vi "AlliGator Define & Save Intensity Corrections File.vi"() -> ()   [LabVIEW 2021, in "AlliGator Intensity Corrections.lvlib"]
doc: "UI to enter intensity correction sepcifications."
uses:
  AlliGator Intensity Corrections.lvlib
  AlliGator Q Element.ctl
  AlliGator Q Event.ctl
  <vilib>/Utility/file.llb/Write Delimited Spreadsheet (DBL).vi
  AlliGator Action Engine.lvlib
panel:
  in  "Save Correction File":bool
  in  "Check Corrections":bool
  out "Intensity Correction":dbl[](graph)
  in  "Acquisition Parameters":string[][](table)=[["1", "1", "550", "200", "250"], ["5", "0.9", "", "", ""], ["15", "0.8", "", "", ""], ["22", "0.7", "", "", ""], ["40", "", "", "", ""], ["53", "", "", "", ""], ["57", "0.6", "", "", ""], ["67", "", "", "", ""], ["73", "", "", "", ""], ["77", "", "", "", ""]]
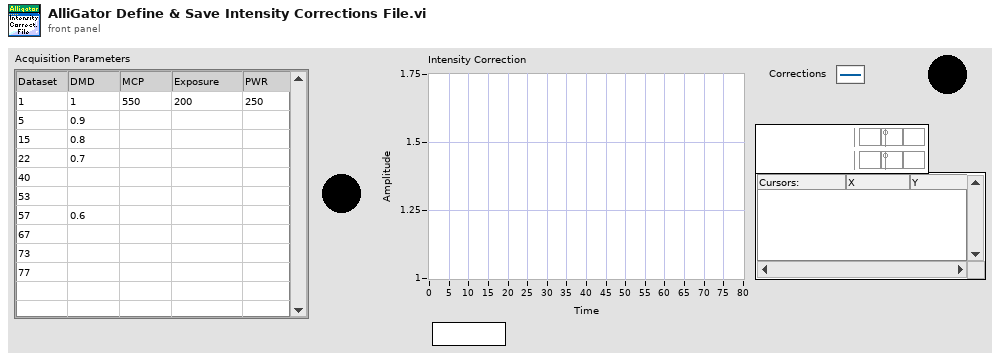
[diagram p1: front panel]
types:
  T1 = typedef "AlliGator Action Engine.lvlib/AlliGator Q Element.ctl" = cluster{"AlliGator Q Event":T2, "Data":variant}
  T2 = typedef "AlliGator Action Engine.lvlib/AlliGator Q Event.ctl" = enum16{"---- Files ----", "Files:Set Batch Export Files To Save", "Files:Set Dataset Loading & Pre-processing Options", "Files:Check #Frames in Dataset", "Files:Increment Frame Index", "Files:Open Mask Image", "Files:Open White Light Image", "Files:Open Single Dataset", "Files:New Folder of Folders Selected", "Files:Load File (all Types)_Scriptable", "Files:Move Flattened Series to Folders Series", "Files:Select Folder", "Files:Load FLI Dataset", "Files:Load Swiss SPAD 1 Dataset", "Files:Load Swiss SPAD 2 Dataset", "Files:Load .sdt FLI Dataset", "Files:Load .ptu FLI Dataset", "Files:Load .bin FLI Dataset", "Files:Load Single Gate Image Folder", "Files:Load I/m/phi Dataset (deprecated)", "Files:Load Single Image", "Files:Subtract Background File", "Files:Export FLI Dataset", "Files:Load HDF5 FLI Dataset", "Files:Set Destination File Path", "Files:Save Mask Image", "Files:Batch Conversion", "Files:New Folder Selected", "Files:Close FLI Dataset", "Files:Close FLI Dataset Series", "Files:Close White Light Image", "Files:Close Mask Image", "---- FLI Dataset ----", "FLI Dataset:Channel Arithmetic", "FLI Dataset:Export Average Lifetime Map as ASCII", "FLI Dataset:Export User-Defined Quantity Map as ASCII", "FLI Dataset:Python Function FLI Dataset Event", "FLI Dataset:ROI Analysis", "FLI Dataset:Tilted Logistic Square Gated IRF Characteristics Map", "FLI Dataset:Logistic Square Gated IRF Characteristics Map", "FLI Dataset:Square Gated IRF Characteristics Map", "FLI Dataset:Multi-ROI Single-Pixel Phasor Analysis", "FLI Dataset:Multi-ROI Single-Pixel NLSF Analysis", "FLI Dataset:All ROIs IRF Extraction", "FLI Dataset:All ROIs Decay Fit Non-Interactive (Fast + Individual IRF)", "FLI Dataset:All ROIs Phasor Analysis", "FLI Dataset:All ROIs Decay Fit", "FLI Dataset:Fluorescence Decay Statistics", "FLI Dataset:Update Decay Statistics Graph", "FLI Dataset:Get Decay from ROI", "FLI Dataset:All ROIs Average Lifetimes", "---- FLI Dataset Series ----", "FLI Dataset Series:Sum All Datasets in Series", "FLI Dataset Series:Add Dataset to Accumulated Dataset", "FLI Dataset Series:Display Accumulated Dataset", "FLI Dataset Series:Clear Dataset Series Sum", "FLI Dataset Series:Time-Series Analysis (NLSF)", "FLI Dataset Series:Time-Series Analysis (Phasor)", "---- Image ----", "Image:Update Image Profile Plots", "Image:Image Histogram Cursor Move", "Image:Image Histogram", "Image:Image Contrast", "Image:Set Image Histogram Cursor Move Flag", "Image:Clear Image Overlay", "Image:Use ROI as Search Area", "Image:Set ROI Diameter", "Image:Save Image Data as TIFF", "Image:Save Displayed Image with Overlay", "Image:Save Image Overlay Only", "Image:Save Image as Hot Pixel Mask", "Image:Change Source Image Color Palette", "Image:Copy Image to Clipboard", "Image:Source Image ROI Selection", "Image:Delete All ROIs", "Image:Delete All Unselected ROIs", "Image:Delete ROI", "Image:Merge All ROIs", "Image:Store ROI", "Image:Source Image ROI Storage", "Image:Export ROI Description to Notebook", "Image:Save ROI", "Image:Load ROI", "Image:Paste ROI Definition", "Image:Clear ROI", "Image:Identify ROIs in Mask Image", "Image:Create Complementary ROI", "Image:Create Contour ROI", "Image:Create ROI(s) from Pixels with Peak above Min_Scriptable", "Image:Create ROI(s) from Pixels with Intensity above Min_Scriptable", "Image:Compute ROI Statistics", "Image:Delete ROI(s) based on ROI Characteristics", "Image:Create ROI Grid", "Image:ROI to Individual Pixel ROIs", "Image:Python Function Source Image Event", "Image:Show Phasor Calibration Map ROI Centers", "Image:Convert ROI to Mask Image", "Image:Mouse Move", "Image:Mouse Up", "Image:Set Source Image Mouse Move Flag", "Image:Add Scale Bar Overlay", "Image:Delete Existing ROIs Option", "---- Decay ----", "Decay:Clear IRF/Reference Plot", "Decay:Clear Local IRFs", "Decay:Add Decay to Graph", "Decay:Smoothen Plot", "Decay:Smoothen Plot Tail", "Decay:Average Selected Plots", "Decay:Extract IRF", "Decay:Optimal IRF Extraction", "Decay:Threshold IRF", "Decay:Fit to Model IRF", "Decay:Fit IRF to Square Gate", "Decay:Fit IRF to Logistic Square Gate", "Decay:Fit IRF to Tilted Logistic Square Gate", "Decay:Create Bounding Cursors Set", "Decay:Export Bounding Cursors Definition to Notebook", "Decay:Denoise Plot", "Decay:Compute Cumulative Function", "Decay:Use as Reference Decay", "Decay:Show Reference Decay/IRF", "Decay:Extrapolate Decay", "Decay:Create Head & Tail Bounding Cursors", "Decay:Store Cursor-defined Head & Tail Fractions", "Decay:Rebin Plot", "Decay:1-Normalize Decay", "Decay:[0-1]-Normalize Plot", "Decay:Straighten Decay", "Decay:Shift Decay", "Decay:Fold Decay", "Decay:Fit Decay", "Decay:Global Fit of Selected Decays", "Decay:Post Global Fit Script", "Decay:Add Global Fit Parameters to Graph", "Decay:Add Decay Parameter(s) to Plot (Graph)", "Decay:Export Decay to Phasor Graph", "Decay:Plot Decay Shifts", "Decay:Compute Average Lifetime", "Decay:Plot Convolution", "Decay:Graph Tip Strip Update", "---- Decay Statistics ----", "Decay Statistics:Tip Strip Update", "---- Intensity Time Trace ----", "Intensity Time Trace:Use File Timestamp", "Intensity Time Trace:Load Intensity Corrections File", "Intensity Time Trace:Clear Intensity Corrections File", "Intensity Time Trace:Tip Strip Update", "---- Phasor Plot ----", "Phasor Plot:Build Phasor Plot", "Phasor Plot:Change Phasor Plot Color Palette", "Phasor Plot:Adjust Phasor Plot Display Range", "Phasor Plot:Highlight Image ROI in Phasor Plot", "Phasor Plot:Save Phasor Plot Image with Overlay", "Phasor Plot:Export Complex Phasor Map", "Phasor Plot:Export Phasor Ratio Map", "Phasor Plot:Export Average Lifetime Map", "Phasor Plot:Compute Phase Lifetime Histogram", "Phasor Plot:Compute Phasor Ratio Histogram", "Phasor Plot:Compute Phase Lifetime vs Intensity Scatter Plot", "Phasor Plot:Weber 2-Component Decomposition", "Phasor Plot:Update Phasor Color Map Vertices", "Phasor Plot:Clear Phasor Overlay", "Phasor Plot:Use Segment Extremities as References", "Phasor Plot:Use UC/Segment Intersections as References", "Phasor Plot:Use UC/Principal Axis Intersections as References", "Phasor Plot:Use UC/Linear Fit Intersections as References", "Phasor Plot:Update Phasor Plot Reference", "Phasor Plot:Show Local Phasor Info in Phasor Plot", "Phasor Plot:Update Phasor Plot State", "Phasor Plot:Phasor Plot ROI Storage", "Phasor Plot:Phasor Plot ROI Selection", "Phasor Plot:Python Function Phasor Plot Event", "Phasor Plot:Overlay Phasor ROI, Ratio or Map in Source Image", "Phasor Plot:Compute Decay of Selected Phasors", "Phasor Plot:Phasor at Image Pixel", "Phasor Plot:Mouse Move", "Phasor Plot:Mouse Up", "Phasor Plot:Display Range Mouse Move", "Phasor Plot:Set Mouse Move Flag", "---- Phasor Graph ----", "Phasor Graph:Calibrated Phasor Map Series", "Phasor Graph:Whole Image Phasor Scatter Plot (Todo)", "Phasor Graph:Get Phasor Value", "Phasor Graph:Create New Phasor Plot Dialog", "Phasor Graph:Update Last Phasor Value", "Phasor Graph:Update Phasor (m, phi)", "Phasor Graph:Remove Single Phasor from Plot", "Phasor Graph:Add Single Phasor to Plot", "Phasor Graph:Remove Phasor Plot", "Phasor Graph:Remove Selected Phasor Plots", "Phasor Graph:Clear Phasor Data", "Phasor Graph:Clear Phasor Graph", "Phasor Graph:Cursor Move", "Phasor Graph:Draw Cursor Connecting Line", "Phasor Graph:Clear Cursor Connecting Line", "Phasor Graph:Find UC Intersection", "Phasor Graph:Use UC/Cursor-Defined Line Intersections", "Phasor Graph:Use Selected Plots Fitted Line/UC Intersections", "Phasor Graph:Use Selected Plots Principal Axis/UC Intersections", "Phasor Graph:Show Single Phasor", "Phasor Graph:Save Single Phasor Plot", "Phasor Graph:Save All Phasor Plots", "Phasor Graph:Load Phasor Plot(s)", "Phasor Graph:Phasor Multiplication", "Phasor Graph:Compute Average Phasor", "Phasor Graph:Compute Multiple Average Phasors (Selected Plots)", "Phasor Graph:Export Single Phasor Plot Phase Lifetimes", "Phasor Graph:Phase Lifetime Trajectory", "Phasor Graph:Phase Lifetime vs Intensity Scatter Plot (deprecated)", "Phasor Graph:Parameter 2 vs Parameter 1 Scatter Plot", "Phasor Graph:Use Cursor n Location", "Phasor Graph:Set Reference n to Current Phase Lifetime Value", "Phasor Graph:Set Reference n to Lifetime Value", "Phasor Graph:Set Cursor n Location", "Phasor Graph:Save Phasor Graph Image", "Phasor Graph:Update SEPL Plot", "Phasor Graph:Export Single Phasor Plot Data", "Phasor Graph:Export Selected Phasor Plots Data", "Phasor Graph:Python Function Phasor Graph Event", "Phasor Graph:Tip Strip Update", "---- Calibration ----", "Calibration:Set Calibration Type", "Calibration:Load/Save Phasor Calibration", "Calibration:Load/Save Phasor Calibration Series", "Calibration:Load/Save Phasor Calibration Map", "Calibration:Use as Calibration", "Calibration:Compute Optimal Calibration from Phasor References", "Calibration:Clear Phasor Calibration", "Calibration:Single Phasor Calibration Information", "Calibration:Use as Calibration Series", "Calibration:Use as Calibration Map", "Calibration:Clear Calibration Series", "Calibration:Phasor Calibration Series Information", "Calibration:Clear Calibration Map", "Calibration:Phasor Calibration Map Information", "Calibration:Apply Phasor Calibration", "Calibration:Update Single Plot Calibration", "Calibration:Update Multiple Plots Calibration", "Calibration:Clear Single Plot Calibration", "Calibration:Clear All Plots Calibrations", "Calibration:Clear Plot(s) Calibration(s)?", "Calibration:Phasor Calibration Maps (# Gates Series)", "---- Phasor Ratio ----", "Phasor Ratio:Clear Reference n", "Phasor Ratio:Toggle Selected Plot(s)  Lock to Reference 1", "Phasor Ratio:Use as Reference n", "Phasor Ratio:Send Reference n to Notebook", "Phasor Ratio:Toggle Selected Plot(s)  Lock to Reference 2", "Phasor Ratio:Compute Phasor Ratio at Mouse Location", "Phasor Ratio:Compute Phasor Plot's Average Phasor Ratio", "Phasor Ratio:Compute Time-Series Phasor Ratios", "Phasor Ratio:Fit Line to Phasor Ratio Plot", "Phasor Ratio:Save References", "Phasor Ratio:Load References", "Phasor Ratio:Update Phasor Reference 1", "Phasor Ratio:Update Phasor Reference 2", "Phasor Ratio:Move Cursor n to Reference n", "Phasor Ratio:Use as Phasor Reference 1 Lifetime", "Phasor Ratio:Use as Phasor Reference 2 Lifetime", "Phasor Ratio:Export Phasor Ratio Map as ASCII", "Phasor Ratio:Tip Strip Update", "---- Lifetime & Other Parameters Graph ----", "Lifetime:Tip Strip Update", "---- Decay Fit Parameter Map ----", "Decay Fit Parameter Map:Export ROI NLSF Data as ASCII", "Decay Fit Parameter Map:Set Decay Fit  Parameter Map Selection", "Decay Fit Parameter Map:Build Decay Fit Parameter Map", "Decay Fit Parameter Map:Change Decay Fit Parameter Map Color Palette", "Decay Fit Parameter Map:Export Decay Fit Parameter Map Data as ASCII", "Decay Fit Parameter Map:Export All Decay Fit Parameter Maps Data as ASCII", "Decay Fit Parameter Map:Send Map Data to Lifetime Graph", "Decay Fit Parameter Map:Save Decay Fit Parameter Map Image", "Decay Fit Parameter Map:Save-Load IRFs & Fit Data", "Decay Fit Parameter Map:Update Local Decay Plots", "Decay Fit Parameter Map:Python Function Decay Fit Parameters Map Event", "Decay Fit Parameter Map:Overlay Decay Fit Parameter Map in Source Image", "Decay Fit Parameter Map:Plot Map Data vs Intensity", "Decay Fit Parameter Map:Mouse Up", "Decay Fit Parameter Map:Display Range Mouse Move", "---- Generic Graph ----", "Generic Graph:Generic XY Graph Event", "Generic Graph:Python Function XY Graph Event", "Generic Graph:New Plot", "Generic Graph:Save Plot", "Generic Graph:XY Plot Histogram", "Generic Graph:Set XY Graph Plot Name", "Generic Graph:Set Last Cursor Style", "Generic Graph:Tip Strip Update", "---- GUI ----", "GUI:Start Script", "GUI:Type of Displayed Image Changed", "GUI:Gate Image Slide Changed", "GUI:Show Busy Icon", "GUI:Show Busy Icon & Abort Button", "GUI:Hide Busy Icon", "GUI:Hide Busy Icon & Abort Button", "GUI:Abort", "GUI:End Script", "GUI:Start Timing", "GUI:End Timing", "GUI:Set State Indicator", "GUI:Send Parameters JSON Strings to Clipboard", "GUI:Set Gate Step", "GUI:Idle", "GUI:Initialization", "GUI:Quit", "GUI:Increment Dataset Index", "GUI:Set Dataset Index to -1", "GUI:Time Series Slider Moved", "GUI:Time Series Slider Changed", "GUI:Toggle Playback or Loop", "GUI:Playback Script", "GUI:Set Phasor Frequency", "GUI:Open Window", "GUI:Start Test Script", "GUI:End Test Script", "DEBUG"}
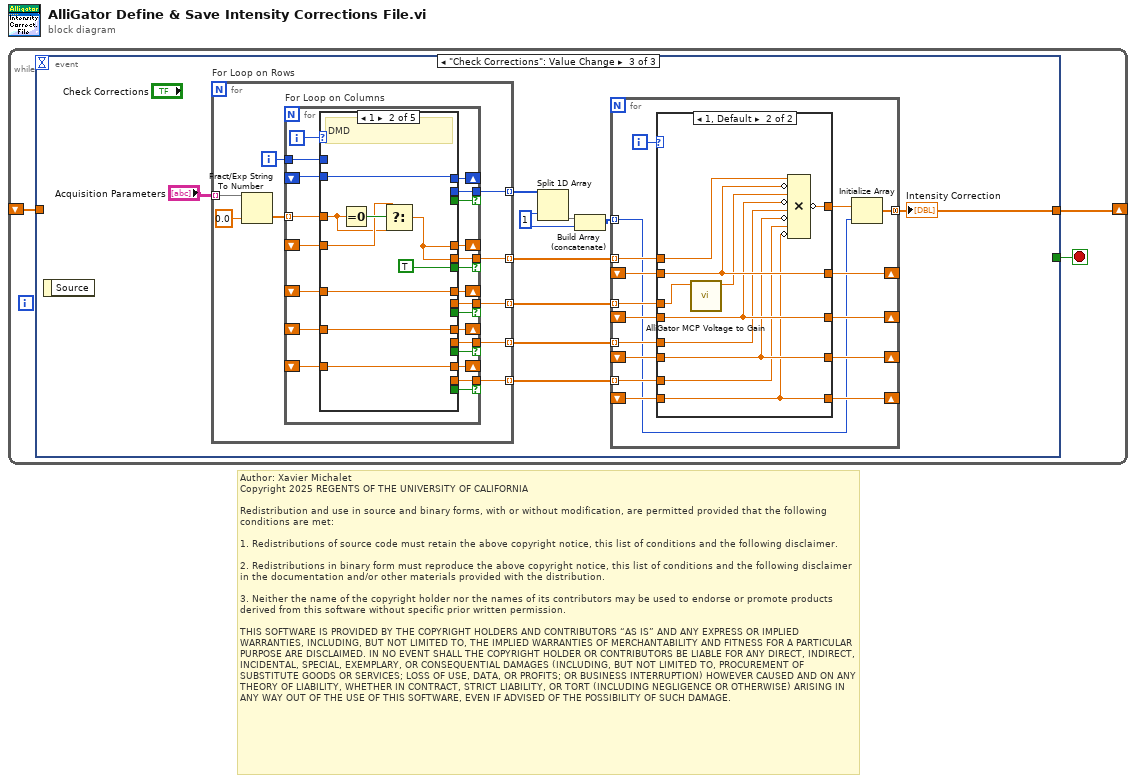
[diagram p0: block diagram]
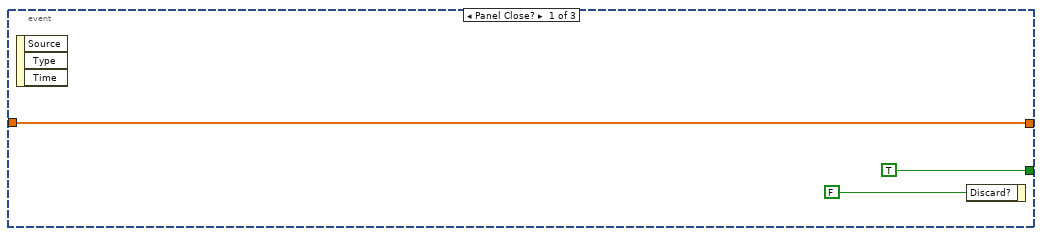
[diagram p2: hidden frame]
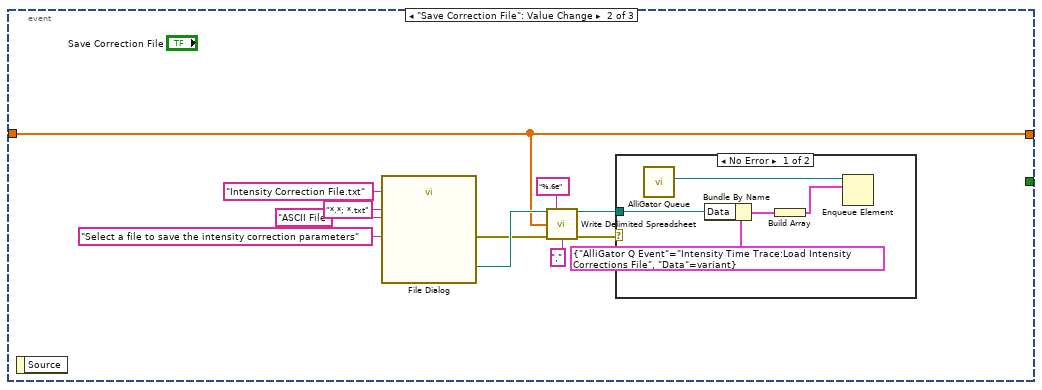
[diagram p3: hidden frame]
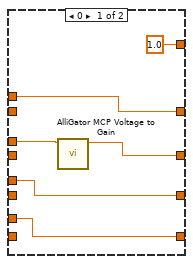
[diagram p5: hidden frame]
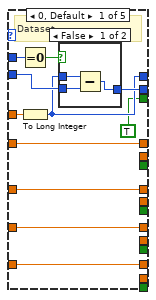
[diagram p6: hidden frame]
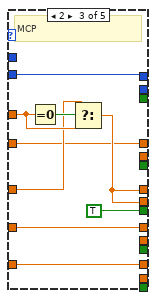
[diagram p8: hidden frame]
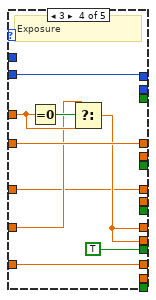
[diagram p9: hidden frame]
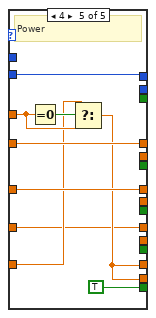
[diagram p10: hidden frame]
diagram:
  # "Author: Xavier Michalet\nCopyright 2025 REGENTS OF THE UNIVERSITY OF CALIFORNIA\n\nRedistribution and use in source and binary forms, with or without modification, are permitted provided that the following conditions are met:\n\n1. Redistributions of source code must retain the above copyright notice, this list of conditions and the following disclaimer.\n\n2. Redistributions in binary form must reproduce the above copyright notice, this list of conditions and the following disclaimer in the documentation and/or other materials provided with the distribution.\n\n3. Neither the name of the copyright holder nor the names of its contributors may be used to endorse or promote products derived from this software without specific prior written permission.\n\nTHIS SOFTWARE IS PROVIDED BY THE COPYRIGHT HOLDERS AND CONTRIBUTORS “AS IS” AND ANY EXPRESS OR IMPLIED WARRANTIES, INCLUDING, BUT NOT LIMITED TO, THE IMPLIED WARRANTIES OF MERCHANTABILITY AND FITNESS FOR A PARTICULAR PURPOSE ARE DISCLAIMED. IN NO EVENT SHALL THE COPYRIGHT HOLDER OR CONTRIBUTORS BE LIABLE FOR ANY DIRECT, INDIRECT, INCIDENTAL, SPECIAL, EXEMPLARY, OR CONSEQUENTIAL DAMAGES (INCLUDING, BUT NOT LIMITED TO, PROCUREMENT OF SUBSTITUTE GOODS OR SERVICES; LOSS OF USE, DATA, OR PROFITS; OR BUSINESS INTERRUPTION) HOWEVER CAUSED AND ON ANY THEORY OF LIABILITY, WHETHER IN CONTRACT, STRICT LIABILITY, OR TORT (INCLUDING NEGLIGENCE OR OTHERWISE) ARISING IN ANY WAY OUT OF THE USE OF THIS SOFTWARE, EVEN IF ADVISED OF THE POSSIBILITY OF SUCH DAMAGE."
  n1 = while {
    shift-right: [w2] -> _
    shift-left: _ -> [w1]
    stop <- w3 stop-if-true
    n2 = event shown="[2] \"Check Corrections\": Value Change" {
      selector: _ -> [_ _ _]
      dyn-events: _ -> [_ _ _]
      timeout: _ -> [_ _ _]
      tunnel: [TRUE _ _] -> w3
      tunnel: [w4 w15 w23] -> w2
      tunnel: w1 -> [w4 w15 _]
      event Panel Close? {
        n3 = event-data() -> ()  [unwired: 1 in, 3 out]
        n4 = event-data("Discard?"=FALSE) -> ()  [unwired: 1 in, 1 out]
      }
      event "Save Correction File": Value Change {
        n5 = event-data() -> ()  [unwired: 1 in, 1 out]
        n6 = call "File Dialog"("prompt"="Select a file to save the intensity correction parameters", "default name"="Intensity Correction File.txt", "pattern (all files)"="*.*; *.txt", "pattern label"="ASCII File") -> ("selected path"=w16:path, "error out"=w14:errorcluster)  [unwired: 8 in, 2 out]
        n7 = call-poly <vilib>:"Write Delimited Spreadsheet.vi"("file path (dialog if empty)"=w16, "format (%.3f)"="%.6e", "1D data"=w15, "error in (no error)"=w14, "delimiter (\\t)"="," ("delimiter (\\t)")) -> ("new file path (Not A Path if cancelled)"=w7:path, "error out"=w8:errorcluster)  [unwired: 9 in]
        n8 = case shown="No Error" w8 {
          tunnel: w7 -> [w20 _]
          frame No Error {
            n9 = call "AlliGator Queue.vi"() -> ("AlliGator Q"=w22:refnum<queue>)  [unwired: 8 in, 1 out]
            n10 = Bundle By Name(cluster=T1 {"AlliGator Q Event"=enum."Intensity Time Trace:Load Intensity Corrections File", "Data"=variant} ("Time-Gated Phasor Q Element"), "Data"=w20) -> (w19:T1)
            n11 = Build Array(w19) -> (w18:T1[])
            n12 = Enqueue Element(queue=w22, element=w18) -> ()  [unwired: 2 in, 3 out]
          }
          frame Error {
          }
        }
      }
      event "Check Corrections": Value Change {
        w32 = 1 ("index")
        n13 = event-data() -> ()  [unwired: 1 in, 1 out]
        n14 = for "For Loop on Rows" {
          tunnel: "Acquisition Parameters" -> [w73] mode=indexing
          tunnel: [w70] -> w26 mode=indexing
          tunnel: [w69] -> w27 mode=indexing
          tunnel: [w68] -> w28 mode=indexing
          tunnel: [w67] -> w29 mode=indexing
          tunnel: [w66] -> w25 mode=indexing
          i -> [w65]
          n15 = Fract/Exp String To Number(string=w73, default (0 dbl)=0.0 ("default (0 I32)")) -> (number=w71:dbl[])  [unwired: 2 in, 1 out]
          n16 = for "For Loop on Columns" {
            tunnel: w71 -> [w95] mode=indexing
            shift-right: [w93] -> _
            shift-left: _ -> [w94]
            shift-right: [w90] -> _
            shift-left: _ -> [w89]
            shift-right: [w84] -> _
            shift-left: _ -> [w86]
            shift-right: [w82] -> _
            shift-left: _ -> [w81]
            tunnel: [w92] -> w70 if=w91
            tunnel: [w88] -> w69 if=w87
            tunnel: [w85] -> w68 if=w83
            tunnel: [w80] -> w67 if=w79
            shift-right: [w77] -> _
            shift-left: _ -> [w78]
            tunnel: [w76] -> w66 if=w74
            tunnel: w65 -> [w75]
            i -> [w96]
            n17 = case shown="1" w96 {
              tunnel: w95 -> [w107 w115 w127 w136 w145]
              tunnel: w94 -> [w106 w118 w123 w135 w144]
              tunnel: [w106 w117 w123 w135 w144] -> w93
              tunnel: [_ w117 _ _ _] -> w92
              tunnel: [_ TRUE _ _ _] -> w91
              tunnel: [w105 w114 w125 w131 w143] -> w90
              tunnel: w89 -> [w105 w114 w126 w131 w143]
              tunnel: [_ _ w125 _ _] -> w88
              tunnel: [_ _ TRUE _ _] -> w87
              tunnel: w86 -> [w104 w113 w122 w134 w139]
              tunnel: [_ _ _ w133 _] -> w85
              tunnel: [w104 w113 w122 w133 w139] -> w84
              tunnel: [_ _ _ TRUE _] -> w83
              tunnel: [w103 w112 w121 w130 w141] -> w82
              tunnel: w81 -> [w103 w112 w121 w130 w142]
              tunnel: [_ _ _ _ w141] -> w80
              tunnel: [_ _ _ _ TRUE] -> w79
              tunnel: w78 -> [w102 w111 w120 w129 w138]
              tunnel: [w101 _ _ _ _] -> w76
              tunnel: [w98 w111 w120 w129 w138] -> w77
              tunnel: w75 -> [w100 _ _ _ _]
              tunnel: [TRUE _ _ _ _] -> w74
              frame 0, Default {
                # "Dataset"
                n18 = Equal To 0?(x=w100) -> (x = 0?=w99:bool)
                n19 = To Long Integer(number=w107) -> (32bit integer=w98:i32)
                n20 = case shown="False" w99 {
                  tunnel: w102 -> [w110 _]
                  tunnel: [w109 _] -> w101
                  tunnel: w98 -> [w108 _]
                  frame False {
                    n21 = Subtract(x=w108, y=w110) -> (x-y=w109:i32)
                  }
                  frame True {
                  }
                }
              }
              frame 1 {
                # "DMD"
                n22 = Equal To 0?(x=w115) -> (x = 0?=w119:bool)
                n23 = Select(t=w118, s=w119, f=w115) -> (s? t:f=w117:dbl)
              }
              frame 2 {
                # "MCP"
                n24 = Equal To 0?(x=w127) -> (x = 0?=w128:bool)
                n25 = Select(t=w126, s=w128, f=w127) -> (s? t:f=w125:dbl)
              }
              frame 3 {
                # "Exposure"
                n26 = Equal To 0?(x=w136) -> (x = 0?=w137:bool)
                n27 = Select(t=w134, s=w137, f=w136) -> (s? t:f=w133:dbl)
              }
              frame 4 {
                # "Power"
                n28 = Equal To 0?(x=w145) -> (x = 0?=w146:bool)
                n29 = Select(t=w142, s=w146, f=w145) -> (s? t:f=w141:dbl)
              }
            }
          }
        }
        n30 = Split 1D Array(array=w25, index=w32) -> (second subarray=w30:i32[])  [unwired: 1 out]
        n31 = Build Array (concatenate)(w30, w32) -> (w31:i32[])
        n32 = for {
          tunnel: w31 -> [w33] mode=indexing
          tunnel: w26 -> [w45] mode=indexing
          tunnel: w27 -> [w43] mode=indexing
          tunnel: w28 -> [w41] mode=indexing
          tunnel: w29 -> [w39] mode=indexing
          tunnel: [w48] -> w23 mode=concatenating
          shift-right: [w46] -> _
          shift-left: _ -> [w38]
          shift-right: [w44] -> _
          shift-left: _ -> [w37]
          shift-right: [w42] -> _
          shift-left: _ -> [w36]
          shift-right: [w40] -> _
          shift-left: _ -> [w35]
          i -> [w47]
          n33 = case shown="1, Default" w47 {
            tunnel: [w54 w62] -> w46
            tunnel: w45 -> [w54 w63]
            tunnel: [w50 w60] -> w44
            tunnel: w43 -> [w51 w64]
            tunnel: [w53 w58] -> w42
            tunnel: w41 -> [w53 w59]
            tunnel: [w52 w56] -> w40
            tunnel: w39 -> [w52 w57]
            tunnel: w38 -> [_ w62]
            tunnel: w37 -> [_ w60]
            tunnel: w36 -> [_ w58]
            tunnel: w35 -> [_ w56]
            tunnel: [1.0 w55] -> w34
            frame 0 {
              n34 = call "AlliGator MCP Voltage to Gain.vi"("MCP Voltage"=w51) -> ("Gain"=w50:dbl)  [unwired: 10 in]
            }
            frame 1, Default {
              n35 = call "AlliGator MCP Voltage to Gain.vi"("MCP Voltage"=w64) -> ("Gain"=w61:dbl)  [unwired: 10 in]
              n36 = Compound Arithmetic op=MULTIPLY(w63, invert w62, w61, invert w60, w59, invert w58, w57, invert w56) -> (invert w55:dbl)
            }
          }
          n37 = Initialize Array(w34, w33) -> (w48:dbl[])
        }
        "Intensity Correction" <- w23
      }
    }
  }
